vi "FROG_read.vi"() -> ()   [LabVIEW 2013]
panel:
  in  "Frequency":path
  in  "Temporal":path
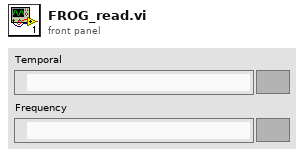
[diagram p1: front panel]
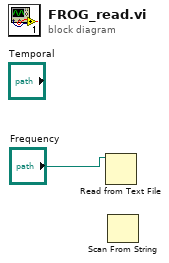
[diagram p0: block diagram]
diagram:
  n1 = Read from Text File(file (use dialog)="Frequency") -> ()  [unwired: 3 in, 4 out]
  n2 = Scan From String() -> ()  [unwired: 5 in, 2 out]
